vi "GUI FOFB Configuration Window.vi"(9 "username":string, 10 "password":string, 11 "FOFB-Controller IP Address in":string="10.0.5.31") -> (3 "Cancelled?":bool)   [LabVIEW 2011, in "User Interface Window VIs.lvlib"]
doc: "Fast Orbit Feedback (FOFB) graphical user interface."
uses:
  User Interface Window VIs.lvlib
  Types Definitions/Type BPM or PS Selector.ctl
  User Interface VIs.lvlib
  XML VIs.lvlib
  Type Definitions.lvlib
panel:
  in  "Refresh Button":bool
  out "Lista de Matrizes Resposta":string[](array[string])
  in  "Response Matrix":string caption="Matriz Resposta Escolhida"
  in  "PS Group ALV":bool
  in  "PS Group ACV":bool
  in  "PS Group ACH":bool
  in  "BPM Selector Vertical":bool
  in  "BPM Selector Horizontal":bool
  in  "PS Graph Selector ALV":T1[](array[typedef]) caption="Grupo ALV"
  in  "PS Graph Selector Vertical":T1[](array[typedef]) caption="Grupo ACV"
  in  "PS Graph Selector Horizontal":T1[](array[typedef]) caption="Grupo ACH"
  in  "BPM Graph Selector Vertical":T1[](array[typedef]) caption="BPMs Verticais"
  in  "BPM Graph Selector Horizontal":T1[](array[typedef]) caption="BPMs Horizontais"
  in  "Cancel Button":bool
  in  "OK Button":bool
  in  "BPM Graph Selector":T1[](array[typedef]) caption="BPMs"
  in  "Vertical (%)":dbl
  in  "Horizontal (%)":dbl
  # "Todos/Nenhum"
  # "Todos/Nenhum"
  # "Todos/Nenhum"
  # "Todos/Nenhum"
  # "Todos/Nenhum"
  # "Fator de correção"
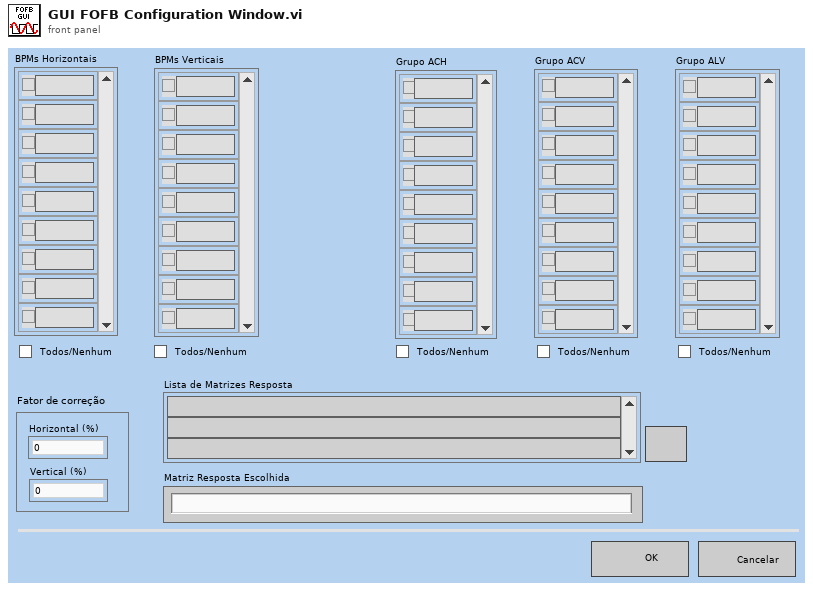
[diagram p1: front panel]
types:
  T1 = typedef "Type Definitions.lvlib/Type BPM or PS Selector.ctl" = cluster{"Name":string, "Active":bool}
  T2 = typedef "Type Definitions.lvlib/Type FOFB Parameters.ctl" = cluster{"Network":T3, "Fast Acquisition":T4, "Response Matrix Measurement":T5, "Correction Algorithm":T6, "Acquisition Network":T7, "Actuation Network":T8}
  T3 = typedef "Type Definitions.lvlib/Type Network Configuration.ctl" = cluster{"FOFB Controller IP":string, "LNLS Control Network IP":string, "LNLS Control Network Power Supplies TCP Port":u16, "LNLS Control Network FOFB Configuration TCP Port":u16, "Data Server TCP Port":u16, "Monitoring Data TCP Port":u16, "Configuration GUI TCP Port":u16, "TCP Listening Timeout":i32}
  T4 = typedef "Type Definitions.lvlib/Type FA Configuration.ctl" = cluster{"Acquisition Period":u32, "Data Buffer Size":u32}
  T5 = typedef "Type Definitions.lvlib/Type Response Matrix Measurement Configuration.ctl" = cluster{"Step Amplitude":dbl, "Time Between Steps":u32, "Step Duration":u32, "Number of Averages":u32}
  T6 = typedef "Type Definitions.lvlib/Type Correction Algorithm Configuration.ctl" = cluster{"Correction Period":u32, "Reference Orbit Path":path, "Response Matrix Path":path, "Correction Matrix Path":path, "Horizontal Correction Factor":dbl, "Vertical Correction Factor":dbl, "Beam Current FOFB Threshold":dbl, "Decouple H-V":bool}
  T7 = typedef "Type Definitions.lvlib/Type Acquisition Network Configuration.ctl" = cluster{"Chassis Name":string, "Variables":cluster{"Variable Name":string, "Matrix Order":u32, "Location":dbl, "Plane":enum8{"H", "V"}, "On Correction":bool}[]}[]
  T8 = typedef "Type Definitions.lvlib/Type Actuation Network Configuration.ctl" = cluster{"Chassis Name":string, "Variables":cluster{"Variable Name":string, "Matrix Order":u32, "RMM Step Factor":dbl, "Plane":enum8{"H", "V"}, "On Correction":bool, "Kc":dbl, "Ti":dbl, "Td":dbl}[]}[]
  T9 = typedef "Type Definitions.lvlib/Type PS Parameters.ctl" = cluster{"RMM Step Factor":dbl, "Plane":enum8{"H", "V"}, "On Correction":bool}
  T10 = typedef "Type Definitions.lvlib/Type BPM Parameters.ctl" = cluster{"Location":dbl, "Plane":enum8{"H", "V"}, "On Correction":bool}
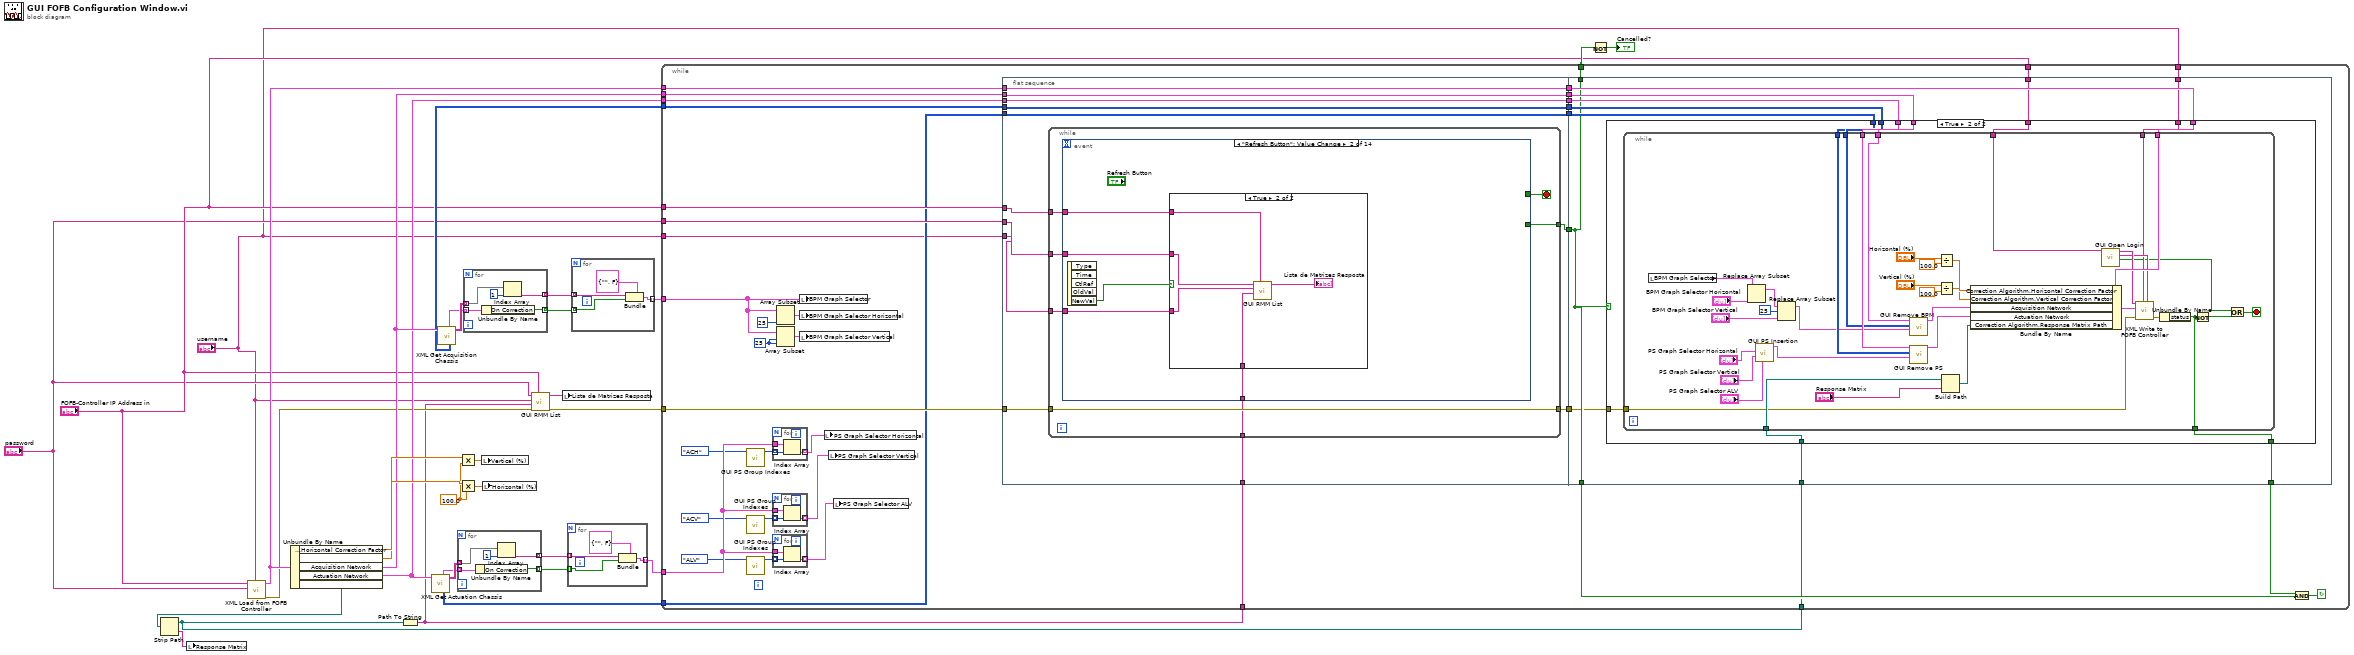
[diagram p0: block diagram]
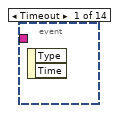
[diagram p2: hidden frame]
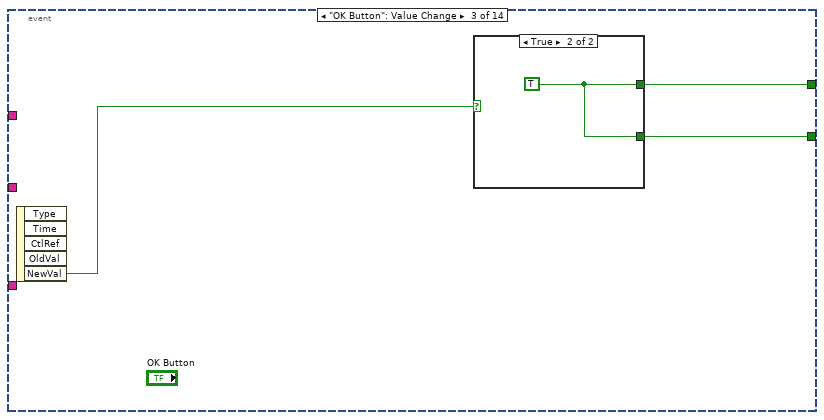
[diagram p4: hidden frame]
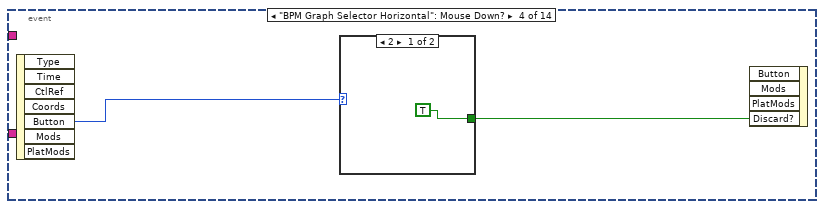
[diagram p6: hidden frame]
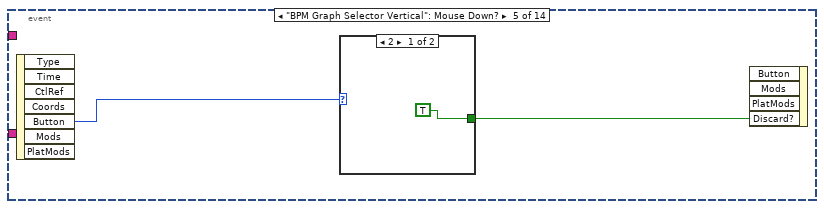
[diagram p8: hidden frame]
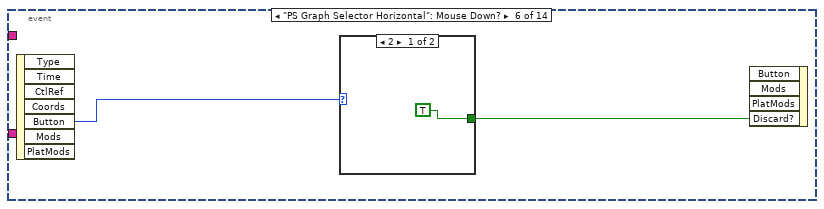
[diagram p10: hidden frame]
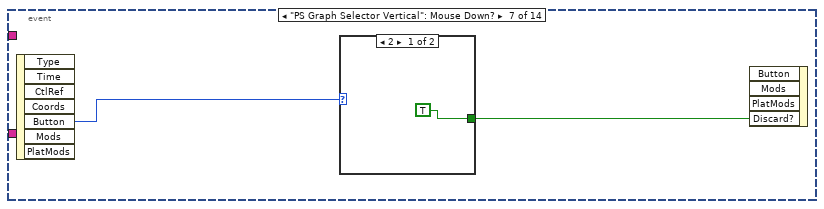
[diagram p12: hidden frame]
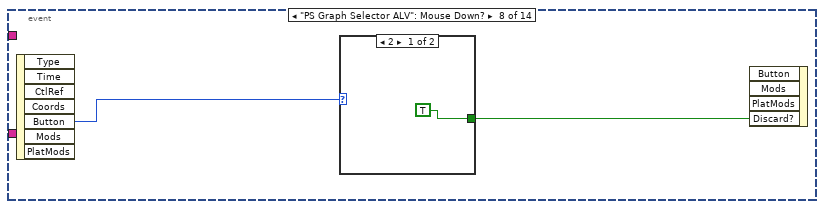
[diagram p14: hidden frame]
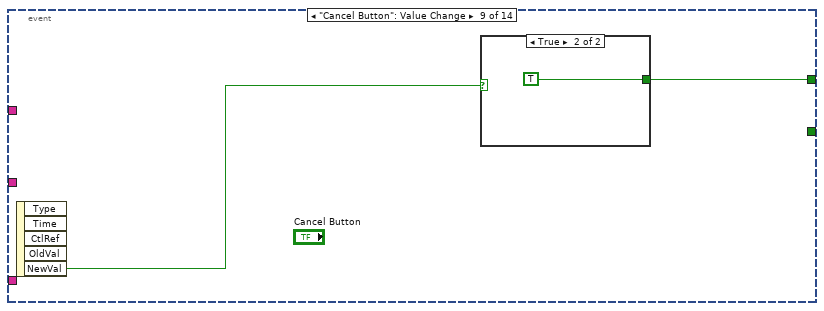
[diagram p16: hidden frame]
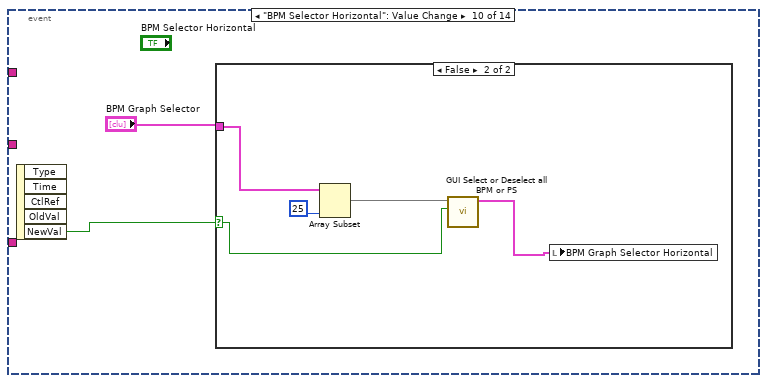
[diagram p18: hidden frame]
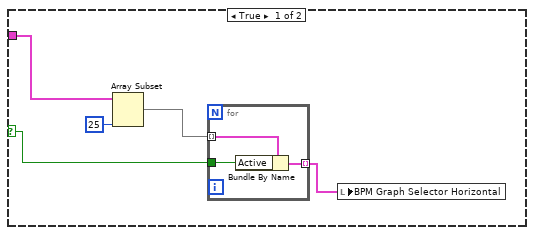
[diagram p19: hidden frame]
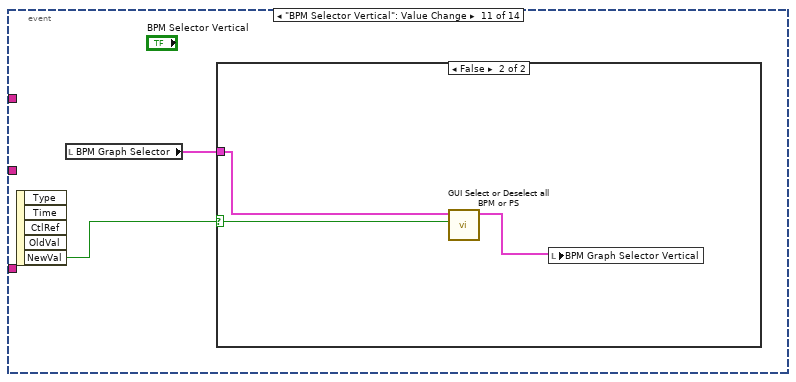
[diagram p20: hidden frame]
diagram:
  w18 = 100.0 ("y")
  n1 = call "XML Load from FOFB Controller.vi"("username"="username", "password"="password", "FOFB-Controller IP Address in"="FOFB-Controller IP Address in") -> ("error out"=w8:errorcluster, "FOFB Parameters"=w17:T2)  [unwired: 7 in]
  n2 = Unbundle By Name(w17) -> ("Correction Algorithm.Horizontal Correction Factor"=w21:dbl, "Correction Algorithm.Vertical Correction Factor"=w20:dbl, "Acquisition Network"=w16:T7, "Actuation Network"=w15:T8, "Correction Algorithm.Response Matrix Path"=w7:path)
  n3 = Strip Path(path=w7) -> (stripped path=w6:path, name=w9:string)
  n4 = local write "Response Matrix"(w9) -> ()
  n5 = Path To String(path=w6) -> (string=w1:string)
  n6 = call "XML Get Actuation Chassis.vi"("Actuation Network"=w15) -> ("Actuation Variable Names"=w27:string[][], "Inverse PS Matrix Mapping"=w13:u32[][], "PS Parameters"=w26:T9[])  [unwired: 3 in, 5 out]
  n7 = call "XML Get Acquisition Chassis.vi"("Acquisition Network"=w16) -> ("Acquisition Variable Names"=w30:string[][], "Inverse BPM Matrix Mapping"=w14:u32[][], "BPM Parameters"=w25:T10[])  [unwired: 4 in, 4 out]
  n8 = for {
    tunnel: w27 -> [w35] mode=indexing
    tunnel: [w34] -> w24 mode=indexing
    tunnel: w26 -> [w33] mode=indexing
    tunnel: [w32] -> w23 mode=indexing
    n9 = Unbundle By Name(w33) -> ("On Correction"=w32:bool)
    n10 = Index Array(array=w35, index=1) -> (element=w34:string)
  }
  n11 = Multiply(x=w20, y=w18) -> (x*y=w19:dbl)
  n12 = Multiply(x=w21, y=w18) -> (x*y=w22:dbl)
  n13 = for {
    tunnel: w30 -> [w40] mode=indexing
    tunnel: [w39] -> w28 mode=indexing
    tunnel: w25 -> [w38] mode=indexing
    tunnel: [w37] -> w29 mode=indexing
    n14 = Unbundle By Name(w38) -> ("On Correction"=w37:bool)
    n15 = Index Array(array=w40, index=1) -> (element=w39:string)
  }
  n16 = local write "Vertical (%)"(w19) -> ()
  n17 = local write "Horizontal (%)"(w22) -> ()
  n18 = call "GUI RMM List.vi"("FOFB-Controller IP Address in"="FOFB-Controller IP Address in", "directory path"=w1, "username"="username", "password"="password") -> ("RMM List"=w5:string[])  [unwired: 6 in, 1 out]
  n19 = local write "Lista de Matrizes Resposta"(w5) -> ()
  n20 = for {
    tunnel: [w44] -> w10 mode=indexing
    tunnel: w23 -> [w42] mode=indexing
    tunnel: w24 -> [w43] mode=indexing
    n21 = Bundle(cluster=T1 {"Name"="", "Active"=FALSE} ("BPM or PS Selection"), "Name"=w43, "Active"=w42) -> (w44:T1)
  }
  n22 = for {
    tunnel: [w48] -> w11 mode=indexing
    tunnel: w29 -> [w46] mode=indexing
    tunnel: w28 -> [w47] mode=indexing
    n23 = Bundle(cluster=T1 {"Name"="", "Active"=FALSE} ("BPM or PS Selection"), "Name"=w47, "Active"=w46) -> (w48:T1)
  }
  n24 = while {
    tunnel: w8 -> [w82]
    tunnel: "FOFB-Controller IP Address in" -> [w81]
    tunnel: "password" -> [w80]
    tunnel: w17 -> [w79]
    tunnel: w16 -> [w78]
    tunnel: w15 -> [w77]
    tunnel: w14 -> [w76]
    tunnel: w13 -> [w75]
    tunnel: [w74] -> w12
    tunnel: w11 -> [w69]
    tunnel: w10 -> [w61]
    tunnel: "FOFB-Controller IP Address in" -> [w65]
    tunnel: "username" -> [w59]
    tunnel: w6 -> [w53]
    tunnel: w1 -> [w52]
    tunnel: "username" -> [w51]
    stop <- w66 continue-if-true
    w71 = 25 ("index")
    n25 = call "GUI PS Group Indexes.vi"("PS Group"=enum16{"ACH", "ACV", "ALV"}."ACH") -> ("Indexes"=w62:i32[])  [unwired: 10 in]
    n26 = call "GUI PS Group Indexes.vi"("PS Group"=enum16{"ACH", "ACV", "ALV"}."ACV") -> ("Indexes"=w58:i32[])  [unwired: 10 in]
    n27 = call "GUI PS Group Indexes.vi"("PS Group"=enum16{"ACH", "ACV", "ALV"}."ALV") -> ("Indexes"=w57:i32[])  [unwired: 10 in]
    n28 = for {
      tunnel: w61 -> [w94]
      tunnel: [w93] -> w64 mode=indexing
      tunnel: w62 -> [w92] mode=indexing
      n29 = Index Array(array=w94, index=w92) -> (element=w93:T1)
    }
    n30 = for {
      tunnel: w61 -> [w97]
      tunnel: [w96] -> w60 mode=indexing
      tunnel: w58 -> [w95] mode=indexing
      n31 = Index Array(array=w97, index=w95) -> (element=w96:T1)
    }
    n32 = for {
      tunnel: w61 -> [w91]
      tunnel: [w90] -> w63 mode=indexing
      tunnel: w57 -> [w89] mode=indexing
      n33 = Index Array(array=w91, index=w89) -> (element=w90:T1)
    }
    n34 = Array Subset(array=w69, length=25) -> (w72:T1[])  [unwired: 1 in]
    n35 = Array Subset(array=w69, index=w71, length=w71) -> (w73:T1[])
    n36 = local write "BPM Graph Selector"(w69) -> ()
    n37 = local write "BPM Graph Selector Horizontal"(w72) -> ()
    n38 = local write "BPM Graph Selector Vertical"(w73) -> ()
    n39 = local write "PS Graph Selector Horizontal"(w64) -> ()
    n40 = local write "PS Graph Selector Vertical"(w60) -> ()
    n41 = local write "PS Graph Selector ALV"(w63) -> ()
    n42 = flat-sequence {
      tunnel: w82 -> [w98]
      tunnel: w81 -> [w102]
      tunnel: w80 -> [w101]
      tunnel: w79 -> [w108]
      tunnel: w78 -> [w107]
      tunnel: w77 -> [w106]
      tunnel: w76 -> [w105]
      tunnel: w75 -> [w104]
      tunnel: [w109] -> w88
      tunnel: [w108] -> w87
      tunnel: [w107] -> w86
      tunnel: [w106] -> w85
      tunnel: [w105] -> w84
      tunnel: [w104] -> w83
      tunnel: w52 -> [w99]
      tunnel: w51 -> [w100]
      tunnel: [w103] -> w50
      tunnel: w88 -> [w213]
      tunnel: w87 -> [w218]
      tunnel: w86 -> [w217]
      tunnel: w85 -> [w216]
      tunnel: w84 -> [w215]
      tunnel: w83 -> [w214]
      tunnel: [w213] -> w74
      tunnel: [w213] -> w67
      tunnel: [w212] -> w68
      tunnel: w65 -> [w211]
      tunnel: w59 -> [w210]
      tunnel: w53 -> [w209]
      tunnel: w50 -> [w208]
      frame #0 {
        n43 = while {
          tunnel: w98 -> [w116]
          tunnel: [w116] -> w103
          tunnel: w101 -> [w114]
          tunnel: w102 -> [w113]
          tunnel: [w112] -> w109
          tunnel: w99 -> [w111]
          tunnel: w100 -> [w110]
          stop <- w115 stop-if-true
          n44 = event shown="[1] \"Refresh Button\": Value Change" {
            selector: _ -> [_ _ _ _ _ _ _ _ _ _ _ _ _ _]
            dyn-events: _ -> [_ _ _ _ _ _ _ _ _ _ _ _ _ _]
            timeout: _ -> [_ _ _ _ _ _ _ _ _ _ _ _ _ _]
            tunnel: [_ _ w129 _ _ _ _ _ w147 _ _ _ _ _] -> w115
            tunnel: w114 -> [_ w119 _ _ _ _ _ _ _ _ _ _ _ _]
            tunnel: w113 -> [_ w118 _ _ _ _ _ _ _ _ _ _ _ _]
            tunnel: [_ _ w128 _ _ _ _ _ _ _ _ _ _ _] -> w112
            tunnel: w111 -> [_ w120 _ _ _ _ _ _ _ _ _ _ _ _]
            tunnel: w110 -> [_ w117 _ _ _ _ _ _ _ _ _ _ _ _]
            event Timeout {
              n45 = event-data() -> ()  [unwired: 1 in, 2 out]
            }
            event "Refresh Button": Value Change {
              n46 = event-data() -> ("NewVal"=w121:bool)  [unwired: 1 in, 4 out]
              n47 = case shown="True" w121 {
                tunnel: w120 -> [_ w122]
                tunnel: w119 -> [_ w124]
                tunnel: w118 -> [_ w125]
                tunnel: w117 -> [_ w123]
                frame False {
                }
                frame True {
                  n48 = call "GUI RMM List.vi"("FOFB-Controller IP Address in"=w125, "directory path"=w122, "username"=w123, "password"=w124) -> ("RMM List"=→"Lista de Matrizes Resposta":string[])  [unwired: 6 in, 1 out]
                }
              }
            }
            event "OK Button": Value Change {
              n49 = event-data() -> ("NewVal"=w127:bool)  [unwired: 1 in, 4 out]
              n50 = case shown="True" w127 {
                tunnel: [_ w130] -> w129
                tunnel: [_ w130] -> w128
                frame False {
                }
                frame True {
                  w130 = TRUE
                }
              }
            }
            event "BPM Graph Selector Horizontal": Mouse Down? {
              n51 = event-data() -> ("Button"=w132:u16)  [unwired: 1 in, 6 out]
              n52 = case shown="2" w132 {
                tunnel: [TRUE ("Discard?") _] -> w131
                frame 2 {
                }
                frame 1, Default {
                }
              }
              n53 = event-data("Discard?"=w131) -> ()  [unwired: 4 in, 1 out]
            }
            event "BPM Graph Selector Vertical": Mouse Down? {
              n54 = event-data() -> ("Button"=w135:u16)  [unwired: 1 in, 6 out]
              n55 = case shown="2" w135 {
                tunnel: [TRUE ("Discard?") _] -> w134
                frame 2 {
                }
                frame 1, Default {
                }
              }
              n56 = event-data("Discard?"=w134) -> ()  [unwired: 4 in, 1 out]
            }
            event "PS Graph Selector Horizontal": Mouse Down? {
              n57 = event-data() -> ("Button"=w138:u16)  [unwired: 1 in, 6 out]
              n58 = case shown="2" w138 {
                tunnel: [TRUE ("Discard?") _] -> w137
                frame 2 {
                }
                frame 1, Default {
                }
              }
              n59 = event-data("Discard?"=w137) -> ()  [unwired: 4 in, 1 out]
            }
            event "PS Graph Selector Vertical": Mouse Down? {
              n60 = event-data() -> ("Button"=w141:u16)  [unwired: 1 in, 6 out]
              n61 = case shown="2" w141 {
                tunnel: [TRUE ("Discard?") _] -> w140
                frame 2 {
                }
                frame 1, Default {
                }
              }
              n62 = event-data("Discard?"=w140) -> ()  [unwired: 4 in, 1 out]
            }
            event "PS Graph Selector ALV": Mouse Down? {
              n63 = event-data() -> ("Button"=w144:u16)  [unwired: 1 in, 6 out]
              n64 = case shown="2" w144 {
                tunnel: [TRUE ("Discard?") _] -> w143
                frame 2 {
                }
                frame 1, Default {
                }
              }
              n65 = event-data("Discard?"=w143) -> ()  [unwired: 4 in, 1 out]
            }
            event "Cancel Button": Value Change {
              n66 = event-data() -> ("NewVal"=w146:bool)  [unwired: 1 in, 4 out]
              n67 = case shown="True" w146 {
                tunnel: [_ TRUE] -> w147
                frame False {
                }
                frame True {
                }
              }
            }
            event "BPM Selector Horizontal": Value Change {
              n68 = event-data() -> ("NewVal"=w150:bool)  [unwired: 1 in, 4 out]
              n69 = case shown="False" w150 {
                selector: w150 -> [w153 w159]
                tunnel: "BPM Graph Selector" -> [w151 w162]
                frame True {
                  n70 = Array Subset(array=w151, length=25) -> (w154:T1[])  [unwired: 1 in]
                  n71 = for {
                    tunnel: w154 -> [w157] mode=indexing
                    tunnel: [w158] -> w152 mode=indexing
                    tunnel: w153 -> [w156]
                    n72 = Bundle By Name(cluster=w157, "Active"=w156) -> (w158:T1)
                  }
                  n73 = local write "BPM Graph Selector Horizontal"(w152) -> ()
                }
                frame False {
                  n74 = Array Subset(array=w162, length=25) -> (w161:T1[])  [unwired: 1 in]
                  n75 = call "GUI Select or Deselect all BPM or PS.vi"("Boolean Value"=w159, "Variable Selector In"=w161) -> ("Variable Selector Out"=w160:T1[])  [unwired: 8 in, 1 out]
                  n76 = local write "BPM Graph Selector Horizontal"(w160) -> ()
                }
              }
            }
            event "BPM Selector Vertical": Value Change {
              n77 = event-data() -> ("NewVal"=w165:bool)  [unwired: 1 in, 4 out]
              n78 = local read "BPM Graph Selector"() -> (w164:T1[])
              n79 = case shown="False" w165 {
                selector: w165 -> [w168 w173]
                tunnel: w164 -> [w166 w174]
                frame True {
                  n80 = for {
                    tunnel: w166 -> [w170] mode=indexing
                    tunnel: [w171] -> w167 mode=indexing
                    tunnel: w168 -> [w169]
                    n81 = Bundle By Name(cluster=w170, "Active"=w169) -> (w171:T1)
                  }
                  n82 = local write "BPM Graph Selector Vertical"(w167) -> ()
                }
                frame False {
                  n83 = call "GUI Select or Deselect all BPM or PS.vi"("Boolean Value"=w173, "Variable Selector In"=w174) -> ("Variable Selector Out"=w172:T1[])  [unwired: 8 in, 1 out]
                  n84 = local write "BPM Graph Selector Vertical"(w172) -> ()
                }
              }
            }
            event "PS Group ACH": Value Change {
              n85 = event-data() -> ("NewVal"=w176:bool)  [unwired: 1 in, 4 out]
              n86 = local read "PS Graph Selector Horizontal"() -> (w175:T1[])
              n87 = case shown="True" w176 {
                selector: w176 -> [w177 w182]
                tunnel: w175 -> [w179 w180]
                frame True {
                  n88 = call "GUI Select or Deselect all BPM or PS.vi"("Boolean Value"=w177, "Variable Selector In"=w179) -> ("Variable Selector Out"=w178:T1[])  [unwired: 8 in, 1 out]
                  n89 = local write "PS Graph Selector Horizontal"(w178) -> ()
                }
                frame False {
                  n90 = for {
                    tunnel: w180 -> [w185] mode=indexing
                    tunnel: [w184] -> w181 mode=indexing
                    tunnel: w182 -> [w183]
                    n91 = Bundle By Name(cluster=w185, "Active"=w183) -> (w184:T1)
                  }
                  n92 = local write "PS Graph Selector Horizontal"(w181) -> ()
                }
              }
            }
            event "PS Group ACV": Value Change {
              n93 = event-data() -> ("NewVal"=w187:bool)  [unwired: 1 in, 4 out]
              n94 = local read "PS Graph Selector Vertical"() -> (w186:T1[])
              n95 = case shown="True" w187 {
                selector: w187 -> [w188 w193]
                tunnel: w186 -> [w190 w191]
                frame True {
                  n96 = call "GUI Select or Deselect all BPM or PS.vi"("Boolean Value"=w188, "Variable Selector In"=w190) -> ("Variable Selector Out"=w189:T1[])  [unwired: 8 in, 1 out]
                  n97 = local write "PS Graph Selector Vertical"(w189) -> ()
                }
                frame False {
                  n98 = for {
                    tunnel: w191 -> [w196] mode=indexing
                    tunnel: [w195] -> w192 mode=indexing
                    tunnel: w193 -> [w194]
                    n99 = Bundle By Name(cluster=w196, "Active"=w194) -> (w195:T1)
                  }
                  n100 = local write "PS Graph Selector Vertical"(w192) -> ()
                }
              }
            }
            event "PS Group ALV": Value Change {
              n101 = event-data() -> ("NewVal"=w198:bool)  [unwired: 1 in, 4 out]
              n102 = local read "PS Graph Selector ALV"() -> (w197:T1[])
              n103 = case shown="False" w198 {
                selector: w198 -> [w199 w204]
                tunnel: w197 -> [w201 w202]
                frame False {
                  n104 = call "GUI Select or Deselect all BPM or PS.vi"("Boolean Value"=w199, "Variable Selector In"=w201) -> ("Variable Selector Out"=w200:T1[])  [unwired: 8 in, 1 out]
                  n105 = local write "PS Graph Selector ALV"(w200) -> ()
                }
                frame True {
                  n106 = for {
                    tunnel: w202 -> [w207] mode=indexing
                    tunnel: [w206] -> w203 mode=indexing
                    tunnel: w204 -> [w205]
                    n107 = Bundle By Name(cluster=w207, "Active"=w205) -> (w206:T1)
                  }
                  n108 = local write "PS Graph Selector ALV"(w203) -> ()
                }
              }
            }
          }
        }
      }
      frame #1 {
        n109 = case shown="True" w213 {
          tunnel: w218 -> [_ w228]
          tunnel: w217 -> [_ w227]
          tunnel: w216 -> [_ w226]
          tunnel: w215 -> [_ w225]
          tunnel: w214 -> [_ w224]
          tunnel: [_ w223] -> w212
          tunnel: w211 -> [_ w222]
          tunnel: w210 -> [_ w221]
          tunnel: w209 -> [_ w220]
          tunnel: w208 -> [_ w219]
          frame False {
          }
          frame True {
            n110 = while {
              tunnel: w228 -> [w265]
              tunnel: w227 -> [w264]
              tunnel: w226 -> [w263]
              tunnel: w225 -> [w262]
              tunnel: w224 -> [w261]
              tunnel: [w232] -> w223
              tunnel: w222 -> [w239]
              tunnel: w221 -> [w236]
              tunnel: w220 -> [w233]
              tunnel: w219 -> [w231]
              stop <- w240 stop-if-true
              n111 = local read "BPM Graph Selector"() -> (w256:T1[])
              n112 = Replace Array Subset(array=w256, new element="BPM Graph Selector Horizontal") -> (w259:T1[])  [unwired: 1 in]
              n113 = call "GUI PS Insertion.vi"("PS Graph Selector ALV"="PS Graph Selector ALV", "PS Graph Selector Vertical"="PS Graph Selector Vertical", "PS Graph Selector Horizontal"="PS Graph Selector Horizontal") -> ("PS Graph Selector out"=w253:T1[])  [unwired: 8 in]
              n114 = Replace Array Subset(array=w259, new element="BPM Graph Selector Vertical", index=25) -> (w255:T1[])
              n115 = call "GUI Remove BPM.vi"("BPM Graph Selector"=w255, "Inverse BPM Matrix Mapping"=w262, "Acquisition Network in"=w264) -> ("Acquisition Network out"=w248:T7)  [unwired: 8 in]
              n116 = call "GUI Remove PS.vi"("PS Graph Selector"=w253, "Inverse PS Matrix Mapping"=w261, "Actuation Network in"=w263) -> ("Actuation Network out"=w247:T8)  [unwired: 8 in]
              n117 = Divide(x="Horizontal (%)", y=100.0) -> (x/y=w243:dbl)
              n118 = Divide(x="Vertical (%)", y=100.0) -> (x/y=w242:dbl)
              n119 = Build Path(base path=w233, name or relative path="Response Matrix") -> (appended path=w235:path)
              n120 = Bundle By Name(cluster=w265, "Correction Algorithm.Horizontal Correction Factor"=w243, "Correction Algorithm.Vertical Correction Factor"=w242, "Acquisition Network"=w248, "Actuation Network"=w247, "Correction Algorithm.Response Matrix Path"=w235) -> (w244:T2)
              n121 = call "GUI Open Login.vi"("FOFB-Controller IP Address in"=w239) -> ("Cancelled?"=w230:bool, "Password"=w237:string, "FOFB-Controller IP Address out"=w238:string)  [unwired: 7 in, 1 out]
              n122 = call "XML Write to FOFB Controller.vi"("Password"=w237, "User"=w236, "error in (no error)"=w231, "FOFB Parameters"=w244, "FOFB-Controller IP Address in"=w238) -> ("error out"=w241:errorcluster)  [unwired: 6 in]
              n123 = Unbundle By Name(w241) -> ("status"=w232:bool)
              n124 = Not(x=w232) -> (.not. x?=w229:bool)
              n125 = Or(x=w230, y=w229) -> (x .or. y?=w240:bool)
            }
          }
        }
      }
    }
    n126 = And(x=w68, y=w67) -> (x .and. y?=w66:bool)
  }
  n127 = Not(x=w12) -> (.not. x?=→"Cancelled?":bool)
